vi "Add Performance Channels.vi"(8 "error in (no error)":errorcluster, 11 "Item Ref in":T1 format="%.0x") -> (0 "error out":errorcluster, 3 "Item Ref out":T1 format="%.0x")   [LabVIEW 2017, in "DSF System Explorer.lvlib"]
uses:
  DSF System Explorer.lvlib
  <vilib>/NI Veristand/Custom Device API/Custom Device Item Ref.ctl
  <vilib>/NI Veristand/Custom Device API/Custom Device Channel.ctl
  <vilib>/NI Veristand/Custom Device API/Custom Device Channel Type.ctl
  <vilib>/NI Veristand/Custom Device API/Custom Device API.lvlib
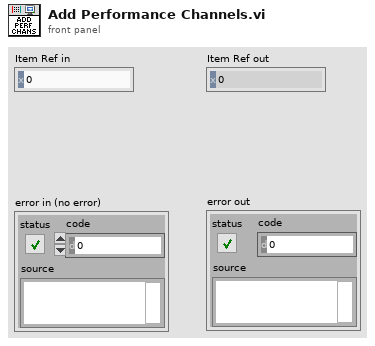
[diagram p1: front panel]
types:
  T1 = typedef "Custom Device API.lvlib/Custom Device Item Ref.ctl" = u64
  T2 = typedef "Custom Device API.lvlib/Custom Device Channel.ctl" = cluster{"Type":T3, "Units":string, "Default Value":dbl, "Faultable":bool, "Scalable":bool}
  T3 = typedef "Custom Device API.lvlib/Custom Device Channel Type.ctl" = enum16{"Input", "Output"}
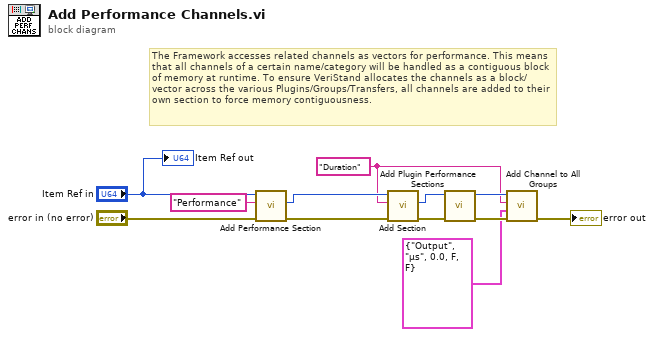
[diagram p0: block diagram]
diagram:
  w1 = "Duration" ("Section Name")
  # "The Framework accesses related channels as vectors for performance. This means that all channels of a certain name/category will be handled as a contiguous block of memory at runtime. To ensure VeriStand allocates the channels as a block/vector across the various Plugins/Groups/Transfers, all channels are added to their own section to force memory contiguousness."
  n1 = call "Add Performance Section.vi"("error in (no error)"="error in (no error)", "Section Name"="Performance", "Item Ref in"="Item Ref in") -> ("error out"=w12:errorcluster, "Performance Section Ptr"=w2:T1)  [unwired: 6 in, 1 out]
  n2 = call "Add Section.vi"("error in (no error)"=w12, "Section Name"=w1, "Item Ref in"=w2) -> ("error out"=w11:errorcluster, "Status Section Ptr"=w10:T1)  [unwired: 6 in, 1 out]
  n3 = call "Add Plugin Performance Sections.vi"("error in (no error)"=w11, "Item Ref in"=w10) -> ("error out"=w8:errorcluster, "Item Ref out"=w9:T1)  [unwired: 8 in]
  n4 = call "Add Channel to All Groups.vi"("error in (no error)"=w8, "Channel"=T2 {"Type"=enum."Output", "Units"="µs", "Default Value"=0.0, "Faultable"=FALSE, "Scalable"=FALSE}, "Channel Name"=w1, "Item Ref in"=w9) -> ("error out"=→"error out":errorcluster)  [unwired: 6 in, 1 out]
  "Item Ref out" <- "Item Ref in"
